vi "Intan_UpdateMarkers_128chan.vi"(0 "Picture In":picture, 1 "ChanSelectMode":u16(ring) items=["A chans (0-31)", "B chans (32-63)", "C chans (64-95)", "D chans (96-127)", "A+B chans (0-63)", "C+D chans 964-127)", "Free Select", "None"], 2 "Amplifier Chans":i32[](listbox)=[1, 4, 13, 14, 15, 16, 17, 22], 3 "plot bounds":T1={"Left"=-911, "Top"=-497, "Right"=196, "Bottom"=275}, 4 "YtxtLabelsAll":string[](array[string])) -> (5 "Picture Out":picture, 6 "update labels":bool)   [LabVIEW 2020]
uses:
  <vilib>/Utility/miscctls.llb/LVRectTypeDef.ctl
panel:
  out "Picture":picture
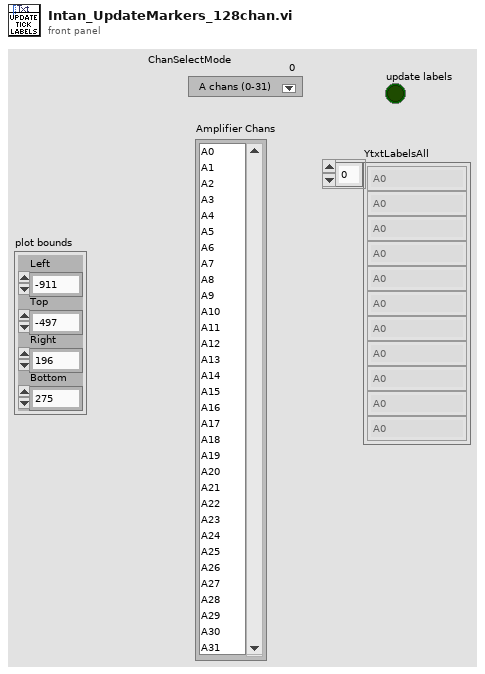
[diagram p1: front panel]
types:
  T1 = typedef "LVRectTypeDef.ctl" = cluster{"Left":i16, "Top":i16, "Right":i16, "Bottom":i16}
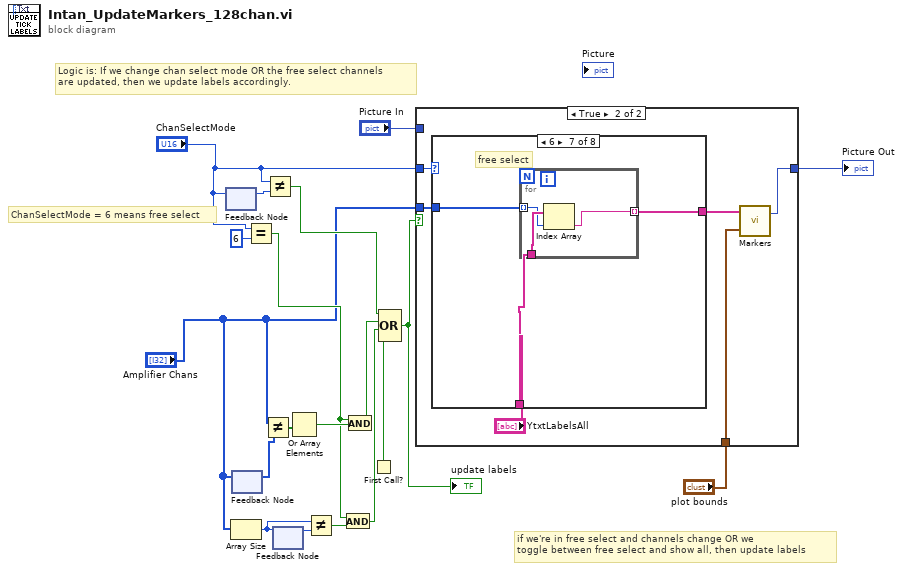
[diagram p0: block diagram]
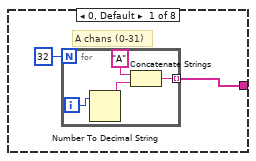
[diagram p3: hidden frame]
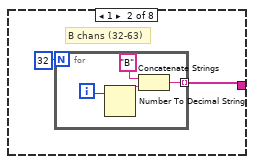
[diagram p4: hidden frame]
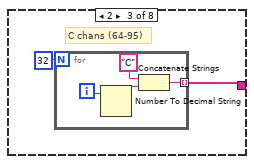
[diagram p5: hidden frame]
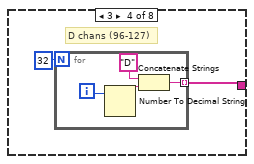
[diagram p6: hidden frame]
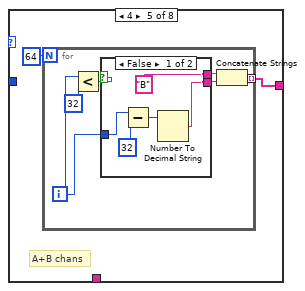
[diagram p7: hidden frame]
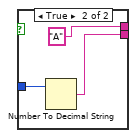
[diagram p8: hidden frame]
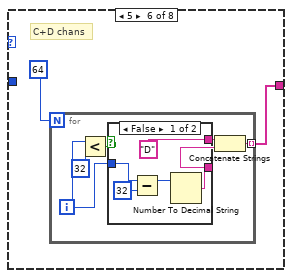
[diagram p9: hidden frame]
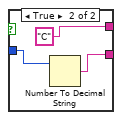
[diagram p10: hidden frame]
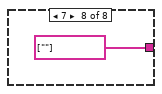
[diagram p11: hidden frame]
diagram:
  # "Logic is: If we change chan select mode OR the free select channels \nare updated, then we update labels accordingly."
  # "ChanSelectMode = 6 means free select"
  # "if we're in free select and channels change OR we\ntoggle between free select and show all, then update labels"
  n1 = feedback #1() -> (w14:u16)  [unwired: 1 in]
  n2 = feedback-in #1("ChanSelectMode") -> ()
  n3 = Array Size(array="Amplifier Chans") -> (size(s)=w13:i32)
  n4 = feedback #2() -> (w18:i32[])  [unwired: 1 in]
  n5 = feedback-in #2("Amplifier Chans") -> ()
  n6 = Equal?(x="ChanSelectMode", y=u16 6) -> (x = y?=w4:bool)
  n7 = Not Equal?(x="Amplifier Chans", y=w18) -> (x != y?=w17:bool[])
  n8 = Not Equal?(x="ChanSelectMode", y=w14) -> (x != y?=w15:bool)
  n9 = feedback #3() -> (w12:i32)  [unwired: 1 in]
  n10 = feedback-in #3(w13) -> ()
  n11 = Or Array Elements(Boolean array=w17) -> (logical OR=w19:bool)
  n12 = Not Equal?(x=w13, y=w12) -> (x != y?=w11:bool)
  n13 = And(x=w4, y=w11) -> (x .and. y?=w10:bool)
  n14 = And(x=w4, y=w19) -> (x .and. y?=w16:bool)
  n15 = First Call?() -> (First Call?: T/F=w9:bool)
  n16 = Compound Arithmetic op=OR(w15, w16, w10, w9) -> (w8:bool)
  "update labels" <- w8
  n17 = case shown="True" w8 {
    tunnel: "ChanSelectMode" -> [_ w25]
    tunnel: "Amplifier Chans" -> [_ w24]
    tunnel: "plot bounds" -> [_ w23]
    tunnel: [w20 w22] -> w6
    tunnel: "Picture In" -> [w20 _]
    frame False {
    }
    frame True {
      n18 = case shown="6" w25 {
        tunnel: w24 -> [_ _ _ _ _ _ w85 _]
        tunnel: [w28 w33 w39 w45 w51 w67 w84 string[] [""]] -> w26
        tunnel: "YtxtLabelsAll" -> [_ _ _ _ _ _ w83 _]
        frame 0, Default {
          # "A chans (0-31)"
          n19 = for {
            N: 32 -> [_]
            tunnel: [w30] -> w28 mode=indexing
            i -> [w29]
            n20 = Number To Decimal String(number=w29) -> (decimal integer string=w32:string)  [unwired: 1 in]
            n21 = Concatenate Strings("A" ("string"), w32) -> (w30:string)
          }
        }
        frame 1 {
          # "B chans (32-63)"
          n22 = for {
            N: 32 -> [_]
            tunnel: [w36] -> w33 mode=indexing
            i -> [w35]
            n23 = Number To Decimal String(number=w35) -> (decimal integer string=w38:string)  [unwired: 1 in]
            n24 = Concatenate Strings("B" ("string"), w38) -> (w36:string)
          }
        }
        frame 2 {
          # "C chans (64-95)"
          n25 = for {
            N: 32 -> [_]
            tunnel: [w42] -> w39 mode=indexing
            i -> [w41]
            n26 = Number To Decimal String(number=w41) -> (decimal integer string=w44:string)  [unwired: 1 in]
            n27 = Concatenate Strings("C" ("string"), w44) -> (w42:string)
          }
        }
        frame 3 {
          # "D chans (96-127)"
          n28 = for {
            N: 32 -> [_]
            tunnel: [w48] -> w45 mode=indexing
            i -> [w47]
            n29 = Number To Decimal String(number=w47) -> (decimal integer string=w50:string)  [unwired: 1 in]
            n30 = Concatenate Strings("D" ("string"), w50) -> (w48:string)
          }
        }
        frame 4 {
          # "A+B chans"
          n31 = for {
            N: 64 -> [_]
            tunnel: [w57] -> w51 mode=indexing
            i -> [w54]
            n32 = Less?(x=w54, y=32) -> (x < y?=w56:bool)
            n33 = case shown="False" w56 {
              tunnel: ["B" ("string") "A" ("string")] -> w58
              tunnel: w54 -> [w61 w65]
              tunnel: [w62 w64] -> w53
              frame False {
                n34 = Subtract(x=w61, y=32) -> (x-y=w60:i32)
                n35 = Number To Decimal String(number=w60) -> (decimal integer string=w62:string)  [unwired: 1 in]
              }
              frame True {
                n36 = Number To Decimal String(number=w65) -> (decimal integer string=w64:string)  [unwired: 1 in]
              }
            }
            n37 = Concatenate Strings(w58, w53) -> (w57:string)
          }
        }
        frame 5 {
          # "C+D chans"
          n38 = for {
            N: 64 -> [_]
            tunnel: [w73] -> w67 mode=indexing
            i -> [w70]
            n39 = Less?(x=w70, y=32) -> (x < y?=w72:bool)
            n40 = case shown="False" w72 {
              tunnel: ["D" ("string") "C" ("string")] -> w74
              tunnel: w70 -> [w78 w81]
              tunnel: [w77 w80] -> w69
              frame False {
                n41 = Subtract(x=w78, y=32) -> (x-y=w76:i32)
                n42 = Number To Decimal String(number=w76) -> (decimal integer string=w77:string)  [unwired: 1 in]
              }
              frame True {
                n43 = Number To Decimal String(number=w81) -> (decimal integer string=w80:string)  [unwired: 1 in]
              }
            }
            n44 = Concatenate Strings(w74, w69) -> (w73:string)
          }
        }
        frame 6 {
          # "free select"
          n45 = for {
            tunnel: w85 -> [w87] mode=indexing
            tunnel: [w86] -> w84 mode=indexing
            tunnel: w83 -> [w88]
            n46 = Index Array(array=w88, index=w87) -> (element=w86:string)
          }
        }
        frame 7 {
        }
      }
      n47 = call "Markers.vi"("plot bounds"=w23, "Array"=w26) -> ("Picture"=w22:picture)  [unwired: 1 out]
    }
  }
  "Picture Out" <- w6
